vi "Read Menu Display Line.vi"(8 "error in (no error)":errorcluster, 11 "VISA resource name":refnum<visa-resource-name>) -> (0 "error out":errorcluster, 2 "Menu Display Line":u8, 3 "VISA resource name out":refnum<visa-resource-name>)   [LabVIEW 2013, in "SRS SR400.lvlib"]
doc: "<B>ML</B>\n\nThe ML command reads the menu line of the display (k in the above table [see Change Menu Display Line.vi]). The ML command is a read only command."
uses:
  <instrlib>/SRS SR400/SRS SR400.lvlib
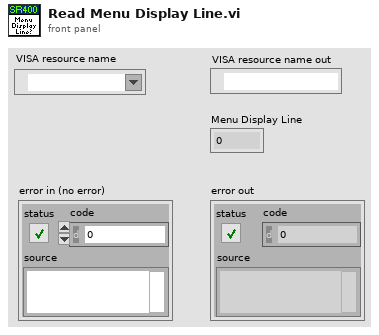
[diagram p1: front panel]
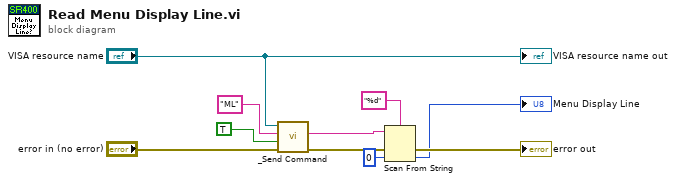
[diagram p0: block diagram]
diagram:
  n1 = call <instrlib>:"_Send Command.vi"("error in (no error)"="error in (no error)", "Read Value? (F)"=TRUE, "Command"="ML" ("command"), "VISA resource name"="VISA resource name") -> ("error out"=w7:errorcluster, "Response"=w8:string)  [unwired: 6 out]
  n2 = Scan From String(format string="%d", input string=w8, error in=w7, default 1=u8 0 ("default value 1")) -> (error out=→"error out":errorcluster, output 1=→"Menu Display Line":u8)  [unwired: 1 in, 2 out]
  "VISA resource name out" <- "VISA resource name"
